vi "Main.vi"   [LabVIEW 2017]
uses:
  TimeTracker.lvclass
  C:/Program Files (x86)/National Instruments/LabVIEW 2017/vi.lib/ActorFramework/Actor/Actor.lvclass
  <vilib>/ActorFramework/Actor/Actor.lvclass
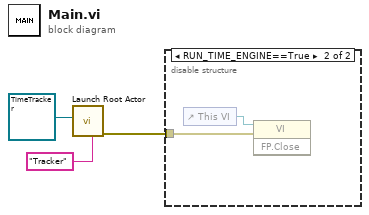
[diagram p0: block diagram]
diagram:
  n1 = call <vilib>:"Launch Root Actor.vi"("Debug Alias"="Tracker", "Actor"=refnum<class "TimeTracker.lvclass"> refnum ("TimeTracker.lvclass")) -> ("error out"=w1:errorcluster)  [unwired: 8 in, 1 out]
  n2 = disable-structure shown="RUN_TIME_ENGINE==True" {
    disable-tunnel: w1 -> [_ w5]
    frame condition #0 (active) {
    }
    frame condition #1 {
      n3 = control-ref of="This VI"() -> (w4:refnum<vi>)
      n4 = invoke class="VI" method="FP.Close"(reference=w4, error in=w5) -> ()  [unwired: 1 in, 3 out]
    }
  }
